vi "cw_functionmaker.vi"(0 "延时选择":i16, 1 "占空比（%）":i8, 2 "初始相位":sgl, 3 "直流偏移":sgl, 5 "停止":bool, 7 "波形选择":enum16{"正弦波", "三角波", "方波", "锯齿波"}(ring), 8 "采样频率（Hz）":sgl, 9 "频率（Hz）":dbl, 10 "幅度（V）":sgl, 11 "采样点数":i32) -> (4 "波形数据":waveform(dbl), 6 "监视器":cluster{i32, sgl, dbl[]}(graph))   [LabVIEW 2022 SP3]
uses:
  <vilib>/Analysis/2dsp.llb/1D Auto Correlation (DBL).vi
  <vilib>/Analysis/NI_AALBase.lvlib
  <vilib>/Analysis/NI_AALPro.lvlib
panel:
  out "自相关 2":dbl[](graph)
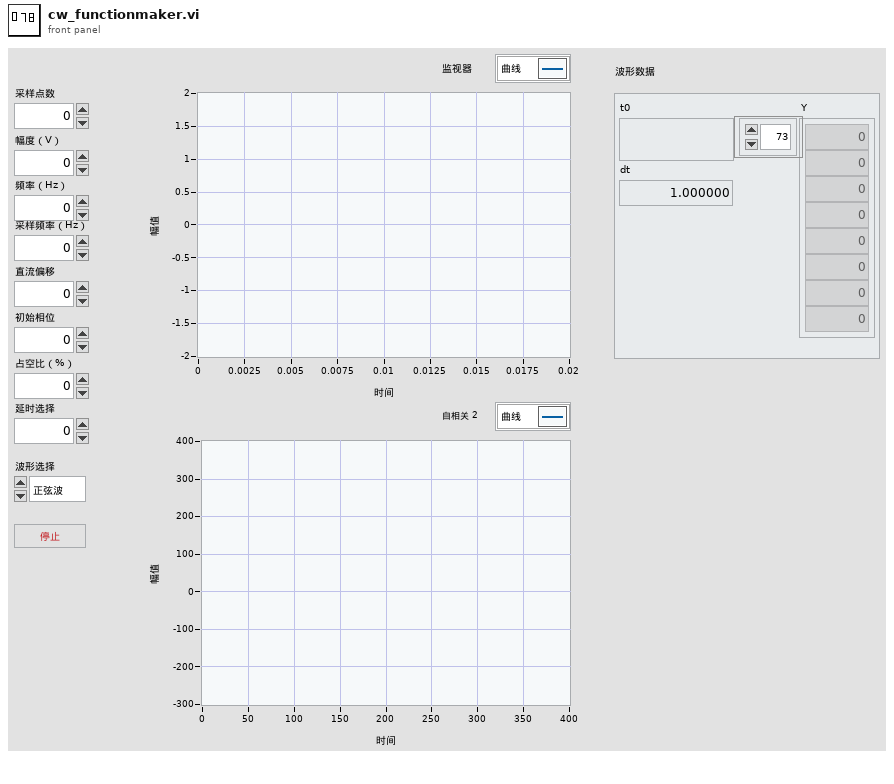
[diagram p1: front panel]
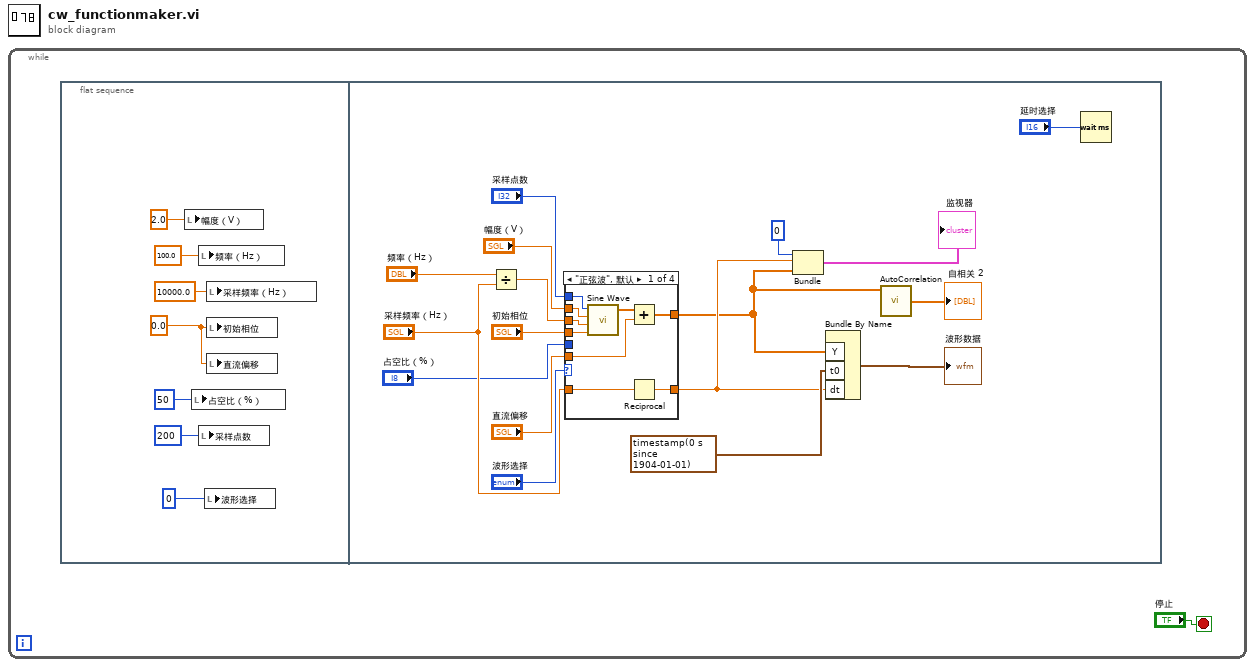
[diagram p0: block diagram]
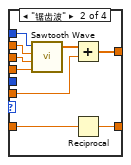
[diagram p2: hidden frame]
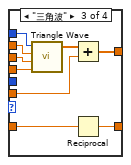
[diagram p3: hidden frame]
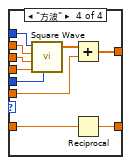
[diagram p4: hidden frame]
diagram:
  n1 = while {
    stop <- "停止" stop-if-true
    n2 = flat-sequence {
      frame #0 {
        w5 = 0.0
        n3 = local write "幅度（V）"(2.0) -> ()
        n4 = local write "占空比（%）"(50) -> ()
        n5 = local write "频率（Hz）"(100.0) -> ()
        n6 = local write "采样点数"(200) -> ()
        n7 = local write "波形选择"(0) -> ()
        n8 = local write "采样频率（Hz）"(10000.0) -> ()
        n9 = local write "初始相位"(w5) -> ()
        n10 = local write "直流偏移"(w5) -> ()
      }
      frame #1 {
        n11 = Divide(x="频率（Hz）", y="采样频率（Hz）") -> (x/y=w16:dbl)
        n12 = case shown="\"正弦波\", 默认" "波形选择" {
          tunnel: "初始相位" -> [w34 w39 w47 w58]
          tunnel: "幅度（V）" -> [w33 w35 w50 w54]
          tunnel: "采样点数" -> [w32 w36 w51 w55]
          tunnel: "采样频率（Hz）" -> [w31 w38 w48 w57]
          tunnel: "直流偏移" -> [w30 w40 w46 w59]
          tunnel: [w28 w42 w44 w60] -> w9
          tunnel: [w27 w41 w45 w61] -> w12
          tunnel: w16 -> [w26 w37 w49 w56]
          tunnel: "占空比（%）" -> [_ _ _ w53]
          frame "正弦波", Default {
            n13 = call <vilib>:"Sine Wave.vi"("samples"=w32, "amplitude"=w33, "frequency"=w26, "phase in"=w34) -> ("sine wave"=w29:dbl[])  [unwired: 1 in, 2 out]
            n14 = Add(x=w29, y=w30) -> (x+y=w28:dbl[])
            n15 = Reciprocal(x=w31) -> (1/x=w27:sgl)
          }
          frame "锯齿波" {
            n16 = call <vilib>:"Sawtooth Wave.vi"("samples"=w36, "amplitude"=w35, "frequency"=w37, "phase in"=w39) -> ("sawtooth wave"=w43:dbl[])  [unwired: 1 in, 2 out]
            n17 = Add(x=w43, y=w40) -> (x+y=w42:dbl[])
            n18 = Reciprocal(x=w38) -> (1/x=w41:sgl)
          }
          frame "三角波" {
            n19 = call <vilib>:"Triangle Wave.vi"("samples"=w51, "amplitude"=w50, "frequency"=w49, "phase in"=w47) -> ("triangle wave"=w52:dbl[])  [unwired: 1 in, 2 out]
            n20 = Add(x=w52, y=w46) -> (x+y=w44:dbl[])
            n21 = Reciprocal(x=w48) -> (1/x=w45:sgl)
          }
          frame "方波" {
            n22 = call <vilib>:"Square Wave.vi"("samples"=w55, "amplitude"=w54, "frequency"=w56, "duty cycle (%)"=w53, "phase in"=w58) -> ("square wave"=w62:dbl[])  [unwired: 1 in, 2 out]
            n23 = Add(x=w62, y=w59) -> (x+y=w60:dbl[])
            n24 = Reciprocal(x=w57) -> (1/x=w61:sgl)
          }
        }
        n25 = Bundle(0, w12, w9) -> (→"监视器":cluster{i32, sgl, dbl[]})  [unwired: 1 in]
        n26 = Bundle By Name("Y"=w9, "t0"=timestamp(0 s since 1904-01-01), "dt"=w12) -> (→"波形数据":waveform(dbl))  [unwired: 1 in]
        n27 = call-poly <vilib>:"AutoCorrelation.vi"("X"=w9) -> ("Rxx"=→"自相关 2":dbl[])  [unwired: 9 in, 1 out]
        n28 = Wait (ms)(milliseconds to wait="延时选择") -> ()  [unwired: 1 out]
      }
    }
  }
